vi "Did Something.vi"(8 "error in (no error)":errorcluster, 10 "Did Something Msg":string) -> (0 "error out":errorcluster)   [LabVIEW 2020, in "Adquisition.lvlib"]
doc: "Send the Did Something event to any VI registered to listen to this module's broadcast events.\n_____\nBased on Delacor QMH Project Template 5.0.0.82."
uses:
  Adquisition.lvlib
  Do Something Argument--cluster.ctl
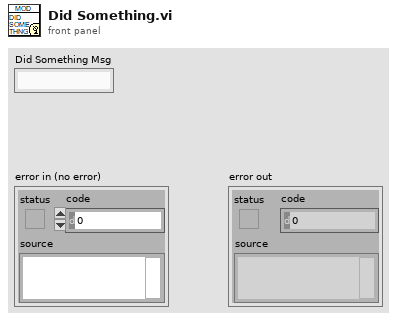
[diagram p1: front panel]
types:
  T1 = typedef "Adquisition.lvlib/Do Something Argument--cluster.ctl" = cluster{"Do Something Msg":string}
  T2 = typedef "Adquisition.lvlib/Broadcast Events--cluster.ctl" = cluster{"Module Did Init":refnum<user-event>, "Status Updated":refnum<user-event>, "Error Reported":refnum<user-event>, "Did Something":refnum<user-event>, "Module Did Stop":refnum<user-event>, "Update Module Execution Status":refnum<user-event>}
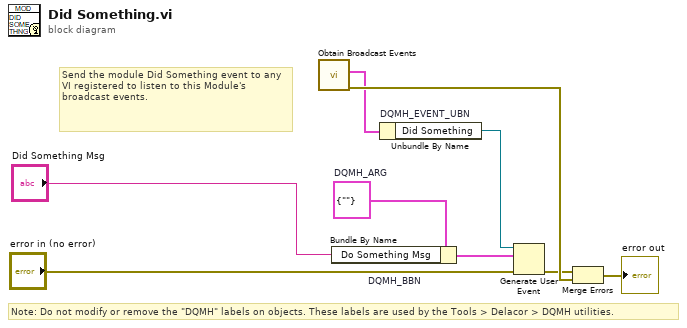
[diagram p0: block diagram]
diagram:
  w3 = T1 {"Do Something Msg"=""}  # DQMH_ARG
  # "Note: Do not modify or remove the \"DQMH\" labels on objects. These labels are used by the Tools > Delacor > DQMH utilities."
  # "Send the module Did Something event to any VI registered to listen to this Module's broadcast events."
  n1 = call "Obtain Broadcast Events.vi"() -> ("error out"=w7:errorcluster, "Adquisition Broadcast Events"=w5:T2)  [unwired: 10 in]
  n2 = Bundle By Name "DQMH_BBN"(cluster=w3, "Do Something Msg"="Did Something Msg") -> (w2:T1)
  n3 = Unbundle By Name "DQMH_EVENT_UBN"(w5) -> ("Did Something"=w4:refnum<user-event>)
  n4 = Generate User Event(user event=w4, event data cluster=w2, error in="error in (no error)") -> (error out=w6:errorcluster)  [unwired: 1 in, 1 out]
  n5 = Merge Errors(w6, w7) -> (→"error out":errorcluster)
